vi "Teardown Error.vi"(7 "Sender":refnum<class "Sender.lvclass">, 11 "Teardown Error in":refnum<class "Teardown Error.lvclass">) -> (3 "Teardown Error out":refnum<class "Teardown Error.lvclass">)   [LabVIEW 2020, in "jettl.lvlib" / "Teardown Error Msg.lvlib" / "Teardown Error.lvclass"]
uses:
  Teardown Error.lvclass
  Sender/Sender/Sender.lvclass
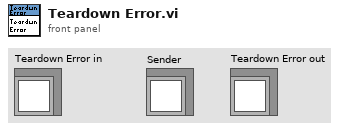
[diagram p1: front panel]
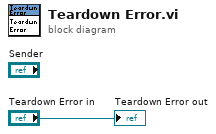
[diagram p0: block diagram]
diagram:
  "Teardown Error out" <- "Teardown Error in"
